vi "RTD_load_preset_list.vi"(7 "relative presets path":string="data\\RTD\\default", 8 "error in":errorcluster, 10 "list in":T1[](array[typedef]) {"tref" format="%.3f"; "Rref [Ohm]" format="%.3f"; "RTD poly" format="%_6e"}, 11 "list ref in":refnum<vi>) -> (0 "error out":errorcluster, 1 "items count":i32, 2 "list out":T1[](array[typedef]) {"tref" format="%.3f"; "Rref [Ohm]" format="%.3f"; "RTD poly" format="%_6e"}, 3 "list ref out":refnum<vi>)   [LabVIEW 2020]
uses:
  RTD_preset.ctl
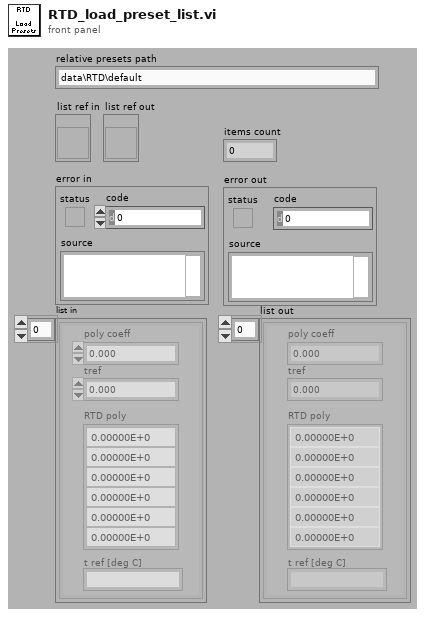
[diagram p1: front panel]
types:
  T1 = typedef "RTD_preset.ctl" = cluster{"Rref [Ohm]":dbl, "tref":dbl, "RTD poly":dbl[], "name":string}
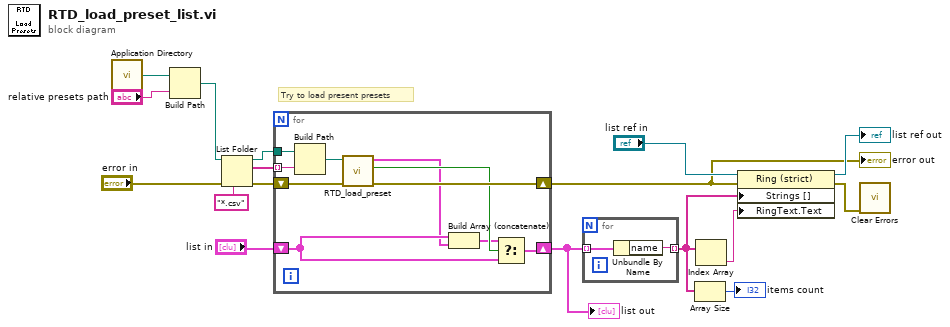
[diagram p0: block diagram]
diagram:
  # "Try to load present presets"
  n1 = call <vilib>:"Application Directory.vi"() -> ("Application Directory"=w17:path)
  n2 = Build Path(base path=w17, name or relative path="relative presets path") -> (appended path=w15:path)
  n3 = List Folder(path=w15, pattern="*.csv", error in="error in") -> (path out=w10:path, filenames=w11:string[], error out=w12:errorcluster)  [unwired: 1 in, 1 out]
  n4 = for {
    shift-right: [w26] -> w4
    shift-left: w12 -> [w27]
    tunnel: w11 -> [w25] mode=indexing
    tunnel: w10 -> [w24]
    shift-right: [w21] -> w9
    shift-left: "list in" -> [w19]
    n5 = Build Path(base path=w24, name or relative path=w25) -> (appended path=w23:path)
    n6 = call "RTD_load_preset.vi"("error in"=w27, "file path"=w23) -> ("error out"=w26:errorcluster, "successfull"=w22:bool, "preset"=w18:T1)  [unwired: 6 in, 1 out]
    n7 = Build Array (concatenate)(w19, w18) -> (w20:T1[])
    n8 = Select(t=w20, s=w22, f=w19) -> (s? t:f=w21:T1[])
  }
  "error out" <- w4
  "list out" <- w9
  n9 = for {
    tunnel: w9 -> [w29] mode=indexing
    tunnel: [w28] -> w2 mode=indexing
    n10 = Unbundle By Name(w29) -> ("name"=w28:string)
  }
  n11 = Array Size(array=w2) -> (size(s)=→"items count":i32)
  n12 = Index Array(array=w2) -> (element=w7:string)  [unwired: 1 in]
  n13 = property class="Ring (strict)"(reference="list ref in", error in=w4, "Strings []"=w2, "RingText.Text"=w7) -> (reference out=→"list ref out":refnum<vi>, error out=w3:errorcluster)
  n14 = call <vilib>:"Clear Errors.vi"("error in (no error)"=w3) -> ()  [unwired: 5 in, 2 out]
